vi "Word Clear by Solution.vi"(11 "Words_Ref in":refnum<vi>[](array[refnum])) -> (3 "Words_Ref out":refnum<vi>[](array[refnum]))   [LabVIEW 2015]
uses:
  TypeDef/Color.ctl
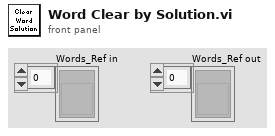
[diagram p1: front panel]
types:
  T1 = enum8{"Enabled", "Disabled", "Disabled and Grayed Out"}
  T2 = typedef "Color.ctl" = u32
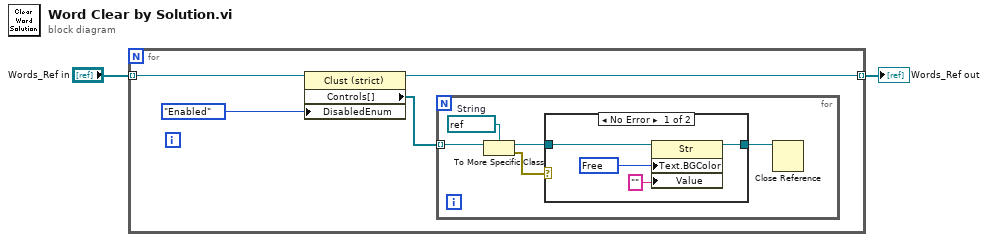
[diagram p0: block diagram]
diagram:
  n1 = for {
    tunnel: "Words_Ref in" -> [w5] mode=indexing
    tunnel: [w4] -> w1 mode=indexing
    n2 = property class="Clust (strict)"(reference=w5, "DisabledEnum"=T1."Enabled" ("Disabled")) -> (reference out=w4:refnum<vi>, "Controls[]"=w6:refnum<vi>[])  [unwired: 1 in, 1 out]
    n3 = for {
      tunnel: w6 -> [w11] mode=indexing
      w9 = refnum<vi> refnum  # String
      n4 = To More Specific Class(target class=w9, reference=w11) -> (specific class reference=w10:refnum<vi>, error out=w8:errorcluster)  [unwired: 1 in]
      n5 = case shown="No Error" w8 {
        tunnel: w10 -> [w15 w16]
        tunnel: [w14 w16] -> w7
        frame No Error {
          w12 = T2 9567230 items=["Free"=9567230, "Letter"=16774186, "Any"=16448250, "Exclude"=12369084] ("Color")
          n6 = property class="Str"(reference=w15, "Text.BGColor"=w12, "Value"="") -> (reference out=w14:refnum<vi>)  [unwired: 1 in, 1 out]
        }
        frame Error {
        }
      }
      n7 = Close Reference(reference=w7) -> ()  [unwired: 1 in, 1 out]
    }
  }
  "Words_Ref out" <- w1
